vi "Swerve Begin.vi"   [LabVIEW 2020]
uses:
  <vilib>/Rock Robotics/SystemInterfaces/AI/FPGA_AIChannel.ctl
  Swerve Global Variables.vi
types:
  T1 = typedef "FPGA_AIChannel.ctl" = enum8{"AI 0", "AI 1", "AI 2", "AI 3", "AI MXP 0", "AI MXP 1", "AI MXP 2", "AI MXP 3", "Invalid"}
  T2 = typedef "WPI_MotorControlDeviceRef.ctl" = cluster{"DeviceStatus":errorcluster, "Type":T3, "PWM":cluster{"PWM Channel":T4, "DeadBand":T5}, "CAN":cluster{"Device Number":u8, "SetOutput VI Ref":variant, "GetOutput VI Ref":variant, "Enable VI Ref":variant, "Disable VI Ref":variant, "Data":variant}, "Invert":bool, "DIO PWM":cluster{"PWM \"Enable\" Channel":T4, "DIOChannel":T6, "PWM Rate":dbl}}
  T3 = typedef "WPI_MotorControlType.ctl" = enum16{"PWM", "CAN", "DIO PWM"}
  T4 = typedef "FPGA_DIOPWMChannel.ctl" = enum8{"PWM 0", "PWM 1", "PWM 2", "PWM 3", "PWM 4", "PWM 5", "PWM 6", "PWM 7", "PWM 8", "PWM 9", "PWM MXP 0", "PWM MXP 1", "PWM MXP 2", "PWM MXP 3", "PWM MXP 4", "PWM MXP 5", "PWM MXP 6", "PWM MXP 7", "PWM MXP 8", "PWM MXP 9", "Invalid"}
  T5 = typedef "WPI_PWMDeadband.ctl" = cluster{"Name":string, "maxPositivePwm":i32, "minPositivePwm":i32, "centerPwm":i32, "maxNegativePwm":i32, "minNegativePwm":i32, "angularRange":u16}
  T6 = typedef "FPGA_DIOChannel.ctl" = enum8{"DIO 0", "DIO 1", "DIO 2", "DIO 3", "DIO 4", "DIO 5", "DIO 6", "DIO 7", "DIO 8", "DIO 9", "DIO MXP 0", "DIO MXP 1", "DIO MXP 2", "DIO MXP 3", "DIO MXP 4", "DIO MXP 5", "DIO MXP 6", "DIO MXP 7", "DIO MXP 8", "DIO MXP 9", "DIO MXP 10", "DIO MXP 11", "DIO MXP 12", "DIO MXP 13", "DIO MXP 14", "DIO MXP 15", "SPI Port CS1", "SPI Port CS2", "SPI Port CS3", "SPI Port MISO", "SPI Port MOSI", "Invalid"}
  T7 = typedef "WPI_AnalogChannelDevRef.ctl" = cluster{"DevStatus":errorcluster, "Analog Channel":T1}
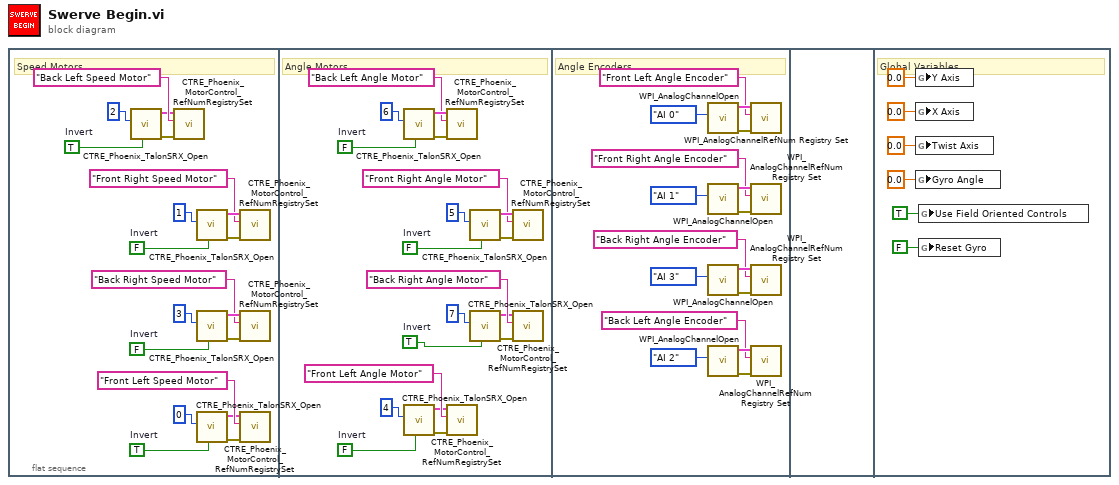
[diagram p0: block diagram]
diagram:
  n1 = flat-sequence "Swerve Initialization" {
    frame #0 {
      w15 = TRUE  # Invert
      w20 = FALSE  # Invert
      w14 = FALSE  # Invert
      w16 = TRUE  # Invert
      # "Speed Motors"
      n2 = call <vilib>:"CTRE_Phoenix_TalonSRX_Open.vi"("Invert"=w15, "Device Number"=u8 2) -> ("error out"=w6:errorcluster, "PhoenixMotorControlDevRef"=w7:T2)  [unwired: 8 in]
      n3 = call <vilib>:"CTRE_Phoenix_MotorControl_RefNumRegistrySet.vi"("error in (no error)"=w6, "refnum name"="Back Left Speed Motor", "PhoenixMotorControlDevRef"=w7) -> ()  [unwired: 7 in, 2 out]
      n4 = call <vilib>:"CTRE_Phoenix_TalonSRX_Open.vi"("Invert"=w14, "Device Number"=u8 1) -> ("error out"=w5:errorcluster, "PhoenixMotorControlDevRef"=w13:T2)  [unwired: 8 in]
      n5 = call <vilib>:"CTRE_Phoenix_TalonSRX_Open.vi"("Invert"=w20, "Device Number"=u8 3) -> ("error out"=w18:errorcluster, "PhoenixMotorControlDevRef"=w19:T2)  [unwired: 8 in]
      n6 = call <vilib>:"CTRE_Phoenix_TalonSRX_Open.vi"("Invert"=w16, "Device Number"=u8 0) -> ("error out"=w8:errorcluster, "PhoenixMotorControlDevRef"=w9:T2)  [unwired: 8 in]
      n7 = call <vilib>:"CTRE_Phoenix_MotorControl_RefNumRegistrySet.vi"("error in (no error)"=w5, "refnum name"="Front Right Speed Motor", "PhoenixMotorControlDevRef"=w13) -> ()  [unwired: 7 in, 2 out]
      n8 = call <vilib>:"CTRE_Phoenix_MotorControl_RefNumRegistrySet.vi"("error in (no error)"=w18, "refnum name"="Back Right Speed Motor", "PhoenixMotorControlDevRef"=w19) -> ()  [unwired: 7 in, 2 out]
      n9 = call <vilib>:"CTRE_Phoenix_MotorControl_RefNumRegistrySet.vi"("error in (no error)"=w8, "refnum name"="Front Left Speed Motor", "PhoenixMotorControlDevRef"=w9) -> ()  [unwired: 7 in, 2 out]
    }
    frame #1 {
      w35 = TRUE  # Invert
      w40 = FALSE  # Invert
      w34 = FALSE  # Invert
      w36 = FALSE  # Invert
      # "Angle Motors"
      n10 = call <vilib>:"CTRE_Phoenix_TalonSRX_Open.vi"("Invert"=w40, "Device Number"=u8 6) -> ("error out"=w38:errorcluster, "PhoenixMotorControlDevRef"=w39:T2)  [unwired: 8 in]
      n11 = call <vilib>:"CTRE_Phoenix_TalonSRX_Open.vi"("Invert"=w36, "Device Number"=u8 4) -> ("error out"=w28:errorcluster, "PhoenixMotorControlDevRef"=w29:T2)  [unwired: 8 in]
      n12 = call <vilib>:"CTRE_Phoenix_MotorControl_RefNumRegistrySet.vi"("error in (no error)"=w38, "refnum name"="Back Left Angle Motor", "PhoenixMotorControlDevRef"=w39) -> ()  [unwired: 7 in, 2 out]
      n13 = call <vilib>:"CTRE_Phoenix_MotorControl_RefNumRegistrySet.vi"("error in (no error)"=w28, "refnum name"="Front Left Angle Motor", "PhoenixMotorControlDevRef"=w29) -> ()  [unwired: 7 in, 2 out]
      n14 = call <vilib>:"CTRE_Phoenix_TalonSRX_Open.vi"("Invert"=w34, "Device Number"=u8 5) -> ("error out"=w25:errorcluster, "PhoenixMotorControlDevRef"=w33:T2)  [unwired: 8 in]
      n15 = call <vilib>:"CTRE_Phoenix_TalonSRX_Open.vi"("Invert"=w35, "Device Number"=u8 7) -> ("error out"=w26:errorcluster, "PhoenixMotorControlDevRef"=w27:T2)  [unwired: 8 in]
      n16 = call <vilib>:"CTRE_Phoenix_MotorControl_RefNumRegistrySet.vi"("error in (no error)"=w25, "refnum name"="Front Right Angle Motor", "PhoenixMotorControlDevRef"=w33) -> ()  [unwired: 7 in, 2 out]
      n17 = call <vilib>:"CTRE_Phoenix_MotorControl_RefNumRegistrySet.vi"("error in (no error)"=w26, "refnum name"="Back Right Angle Motor", "PhoenixMotorControlDevRef"=w27) -> ()  [unwired: 7 in, 2 out]
    }
    frame #2 {
      # "Angle Encoders"
      n18 = call <vilib>:"WPI_AnalogChannelOpen.vi"("Analog Channel"=FPGA_AIChannel."AI 0") -> ("error out"=w50:errorcluster, "AIDeviceRef"=w49:T7)  [unwired: 9 in]
      n19 = call <vilib>:"WPI_AnalogChannelOpen.vi"("Analog Channel"=FPGA_AIChannel."AI 1") -> ("error out"=w52:errorcluster, "AIDeviceRef"=w51:T7)  [unwired: 9 in]
      n20 = call <vilib>:"WPI_AnalogChannelOpen.vi"("Analog Channel"=FPGA_AIChannel."AI 3") -> ("error out"=w56:errorcluster, "AIDeviceRef"=w55:T7)  [unwired: 9 in]
      n21 = call <vilib>:"WPI_AnalogChannelOpen.vi"("Analog Channel"=FPGA_AIChannel."AI 2") -> ("error out"=w54:errorcluster, "AIDeviceRef"=w53:T7)  [unwired: 9 in]
      n22 = call <vilib>:"WPI_AnalogChannelRefNum Registry Set.vi"("error in (no error)"=w50, "refnum name"="Front Left Angle Encoder", "AIDeviceRef"=w49) -> ()  [unwired: 7 in, 2 out]
      n23 = call <vilib>:"WPI_AnalogChannelRefNum Registry Set.vi"("error in (no error)"=w52, "refnum name"="Front Right Angle Encoder", "AIDeviceRef"=w51) -> ()  [unwired: 7 in, 2 out]
      n24 = call <vilib>:"WPI_AnalogChannelRefNum Registry Set.vi"("error in (no error)"=w56, "refnum name"="Back Right Angle Encoder", "AIDeviceRef"=w55) -> ()  [unwired: 7 in, 2 out]
      n25 = call <vilib>:"WPI_AnalogChannelRefNum Registry Set.vi"("error in (no error)"=w54, "refnum name"="Back Left Angle Encoder", "AIDeviceRef"=w53) -> ()  [unwired: 7 in, 2 out]
    }
    frame #3 {
    }
    frame #4 {
      # "Global Variables"
      n26 = global write "Swerve Global Variables.vi" "Y Axis"(0.0 ("Y Axis")) -> ()
      n27 = global write "Swerve Global Variables.vi" "X Axis"(0.0 ("X Axis")) -> ()
      n28 = global write "Swerve Global Variables.vi" "Twist Axis"(0.0 ("Twist Axis")) -> ()
      n29 = global write "Swerve Global Variables.vi" "Gyro Angle"(0.0 ("Gyro Angle")) -> ()
      n30 = global write "Swerve Global Variables.vi" "Use Field Oriented Controls"(TRUE ("Use Field Oriented Controls")) -> ()
      n31 = global write "Swerve Global Variables.vi" "Reset Gyro"(FALSE ("Reset Gyro")) -> ()
    }
  }
